vi "Configure RT Noise.vi"(0 "VISA resource name":refnum<visa-resource-name>, 1 "Enable Noise (F:Disable)":bool, 5 "Modulation Format (1: Dual Modulation)":u16(ring)=1 items=["Dual Modulation"=1, "Dual ARB"=2, "Multitone"=3, "Two-tone"=6], 7 "Carrier Bandwidth (1 Hz)":dbl=1.0, 9 "Noise Bandwidth (1 Hz)":dbl=1.0, 11 "error in (no error)":errorcluster, 12 "Noise Bandwidth Factor (1)":u16(ring)=1 items=["1"=1, "2"=2], 13 "Noise Ratio (0 dB)":dbl) -> (4 "VISA resource name out":refnum<visa-resource-name>, 15 "error out":errorcluster)   [LabVIEW 2014, in "Agilent PSG MXG Series.lvlib"]
doc: "Configures real-time additive white gaussian noise (AWGN) added to the carrier.\n\n<B>Notes:</B>\n(1) This VI is valid only in E8267D, N5162A, N5182A, N5172B, N5182B.\n\n(2) For E8267D, this VI is valid only when the instrument installs <B>Option 601</B> or <B>Option 602</B> (Internal baseband generator), and <B>Option 403</B> (Calibrated noise, AWGN).\n\n(3) For N5162A and N5182A, this VI is valid only when the instrument installs <B>Option 403</B> (Calibrated noise, AWGN).\n\n(4) For N5172B and N5182B, this VI is valid only when the instrument installs <B>Option 403</B> (Calibrated noise, AWGN)."
uses:
  Agilent PSG MXG Series.lvlib
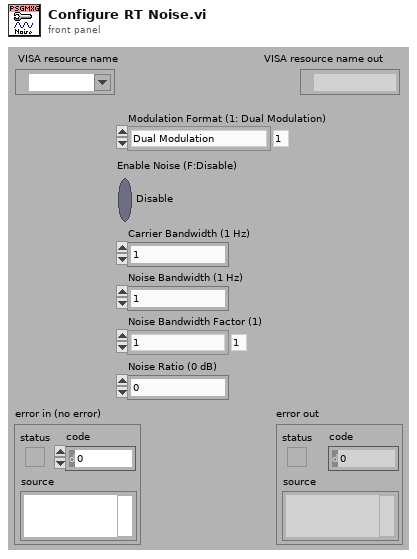
[diagram p1: front panel]
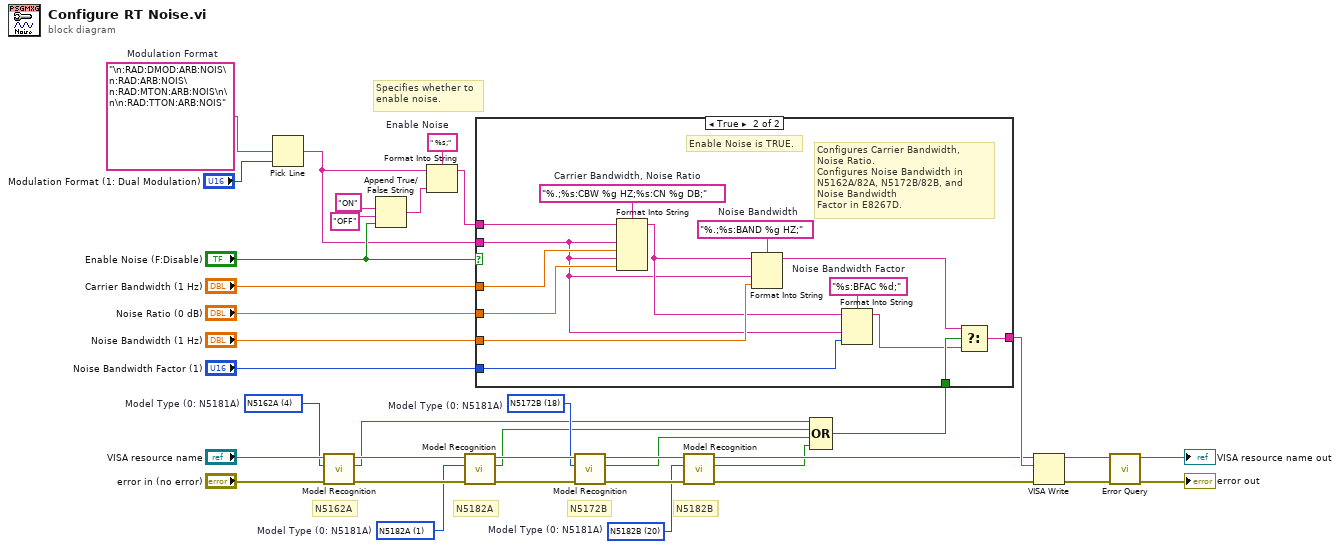
[diagram p0: block diagram]
diagram:
  w5 = u16 20 items=["N5181A"=0, "N5182A"=1, "N5183A"=2, "N5161A"=3, "N5162A"=4, "E8241A"=5, "E8244A"=6, "E8251A"=7, "E8254A"=8, "E8247C"=10, "E8257C"=11, "E8267C"=12, "E8257D"=15, "E8267D"=16, "N5171B"=17, "N5172B"=18, "N5181B"=19, "N5182B"=20]  # Model Type (0: N5181A)
  w3 = u16 18 items=["N5181A"=0, "N5182A"=1, "N5183A"=2, "N5161A"=3, "N5162A"=4, "E8241A"=5, "E8244A"=6, "E8251A"=7, "E8254A"=8, "E8247C"=10, "E8257C"=11, "E8267C"=12, "E8257D"=15, "E8267D"=16, "N5171B"=17, "N5172B"=18, "N5181B"=19, "N5182B"=20]  # Model Type (0: N5181A)
  w8 = u16 4 items=["N5181A"=0, "N5182A"=1, "N5183A"=2, "N5161A"=3, "N5162A"=4, "E8241A"=5, "E8244A"=6, "E8251A"=7, "E8254A"=8, "E8247C"=10, "E8257C"=11, "E8267C"=12, "E8257D"=15, "E8267D"=16, "N5171B"=17, "N5172B"=18, "N5181B"=19, "N5182B"=20]  # Model Type (0: N5181A)
  w9 = u16 1 items=["N5181A"=0, "N5182A"=1, "N5183A"=2, "N5161A"=3, "N5162A"=4, "E8241A"=5, "E8244A"=6, "E8251A"=7, "E8254A"=8, "E8247C"=10, "E8257C"=11, "E8267C"=12, "E8257D"=15, "E8267D"=16, "N5171B"=17, "N5172B"=18, "N5181B"=19, "N5182B"=20]  # Model Type (0: N5181A)
  w35 = " %s;"  # Enable Noise
  w37 = "\n:RAD:DMOD:ARB:NOIS\n:RAD:ARB:NOIS\n:RAD:MTON:ARB:NOIS\n\n\n:RAD:TTON:ARB:NOIS"  # Modulation Format
  # "N5172B"
  # "N5182B"
  # "N5182A"
  # "N5162A"
  # "Specifies whether to\nenable noise."
  # "N5182A"
  n1 = Pick Line(multi-line string=w37, line index="Modulation Format (1: Dual Modulation)") -> (output string=w29:string)  [unwired: 1 out]
  n2 = call "Model Recognition.vi"("error in (no error)"="error in (no error)", "Model Type (0: N5181A)"=w8, "VISA resource name"="VISA resource name") -> ("error out"=w16:errorcluster, "Is Model Correct"=w1:bool, "VISA resource name out"=w18:refnum<visa-resource-name>)  [unwired: 6 out]
  n3 = Append True/False String(1:"Enable Noise (F:Disable)", 2:"OFF" ("false string"), 3:"ON" ("true string")) -> (0:w34:string)  [unwired: 1 out]
  n4 = Format Into String(format string=w35, initial string=w29, w34) -> (resulting string=w30:string)  [unwired: 1 in, 1 out]
  n5 = call "Model Recognition.vi"("error in (no error)"=w16, "Model Type (0: N5181A)"=w9, "VISA resource name"=w18) -> ("error out"=w14:errorcluster, "Is Model Correct"=w2:bool, "VISA resource name out"=w15:refnum<visa-resource-name>)  [unwired: 6 out]
  n6 = call "Model Recognition.vi"("error in (no error)"=w14, "Model Type (0: N5181A)"=w3, "VISA resource name"=w15) -> ("error out"=w12:errorcluster, "Is Model Correct"=w4:bool, "VISA resource name out"=w13:refnum<visa-resource-name>)  [unwired: 6 out]
  n7 = call "Model Recognition.vi"("error in (no error)"=w12, "Model Type (0: N5181A)"=w5, "VISA resource name"=w13) -> ("error out"=w10:errorcluster, "Is Model Correct"=w6:bool, "VISA resource name out"=w11:refnum<visa-resource-name>)  [unwired: 6 out]
  n8 = Compound Arithmetic op=OR(w1, w2, w4, w6) -> (w7:bool)
  n9 = case shown="True" "Enable Noise (F:Disable)" {
    tunnel: w30 -> [w38 w52]
    tunnel: w29 -> [_ w44]
    tunnel: "Carrier Bandwidth (1 Hz)" -> [_ w50]
    tunnel: "Noise Ratio (0 dB)" -> [_ w49]
    tunnel: [w38 w39] -> w22
    tunnel: "Noise Bandwidth (1 Hz)" -> [_ w47]
    tunnel: "Noise Bandwidth Factor (1)" -> [_ w43]
    tunnel: w7 -> [_ w42]
    frame False {
      # "Enable Noise is FALSE."
    }
    frame True {
      w46 = "%s:BFAC %d;"  # Noise Bandwidth Factor
      w48 = "%.;%s:BAND %g HZ;"  # Noise Bandwidth
      w51 = "%.;%s:CBW %g HZ;%s:CN %g DB;"  # Carrier Bandwidth, Noise Ratio
      # "Configures Carrier Bandwidth,\nNoise Ratio.\nConfigures Noise Bandwidth in\nN5162A/82A, N5172B/82B, and Noise Bandwidth\nFactor in E8267D."
      # "Enable Noise is TRUE."
      n10 = Format Into String(format string=w51, initial string=w52, w44, w50, w44, w49) -> (resulting string=w45:string)  [unwired: 1 in, 1 out]
      n11 = Format Into String(format string=w48, initial string=w45, w44, w47) -> (resulting string=w41:string)  [unwired: 1 in, 1 out]
      n12 = Format Into String(format string=w46, initial string=w45, w44, w43) -> (resulting string=w40:string)  [unwired: 1 in, 1 out]
      n13 = Select(t=w41, s=w42, f=w40) -> (s? t:f=w39:string)
    }
  }
  n14 = VISA Write(VISA resource name=w11, write buffer=w22, error in (no error)=w10) -> (VISA resource name out=w26:refnum<visa-resource-name>, error out=w25:errorcluster)  [unwired: 1 out]
  n15 = call "Error Query.vi"("error in (no error)"=w25, "VISA resource name"=w26) -> ("error out"=→"error out":errorcluster, "VISA resource name out"=→"VISA resource name out":refnum<visa-resource-name>)  [unwired: 8 out]
